vi "Utility - Configuration File Generator.vi"() -> ()   [LabVIEW 2013]
uses:
  controls/TDMS Properties.ctl
  controls/Acquisition and Logging Configuration.ctl
  <vilib>/Utility/xml.llb/Write to XML File(string).vi
panel:
  in  "Enable Time Trigger":bool caption="启用时间触发"
  in  "Enable RMS Trigger":bool=TRUE caption="启用RMS触发"
  in  "Log Continuously":bool caption="连续记录"
  in  "TDMS Properties":T1[](array[typedef])=[{"Name"="公司", "Value"="[公司名称]"}, {"Name"="作者(author)", "Value"="[开发者姓名]"}, {"Name"="运算符", "Value"="[操作员名]"}, {"Name"="测试系统", "Value"="[系统名]"}, {"Name"="位置", "Value"="[位置]"}, {"Name"="线", "Value"="[行]"}, {"Name"="机器", "Value"="[机器名]"}, {"Name"="说明", "Value"="[说明]"}] caption="TDMS属性"
  in  "Trigger - Time (Minute)":i32=30 caption="触发－时间（分钟）"
  in  "Trigger - Channel":i32 caption="触发－通道"
  in  "Trigger - RMS Value":dbl=2.0 caption="触发－均方根值"
  in  "Channel Names":string[](array[string])=["Dev1/ai0", "Dev1/ai1", "Dev1/ai2", "Dev1/ai3"] caption="通道名"
  in  "Channel Scale Array":dbl[](array[numeric])=[1.0, 1.0, 1.0, 1.0] caption="通道换算数组"
  in  "Number of Channels":i32=4 caption="通道数"
  in  "Data File Name":string="DAQ_数据" caption="数据文件名"
  in  "Number of Reads to Save":i32=20 caption="用于保存的读取次数"
  in  "Samples per Read":i32=1000 caption="每次读取采样"
  in  "Data Rate (Hz)":dbl=1000.0 caption="数据率(Hz)"
  # "操作步骤：为下列控件赋值，然后运行VI，在项目的根目录中生成Config.xml文件。\n\n注：生成Config.xml以后，需将其复制至RT终端根目录中。"
  # "采集"
  # "通道"
  # "记录"
  # "触发"
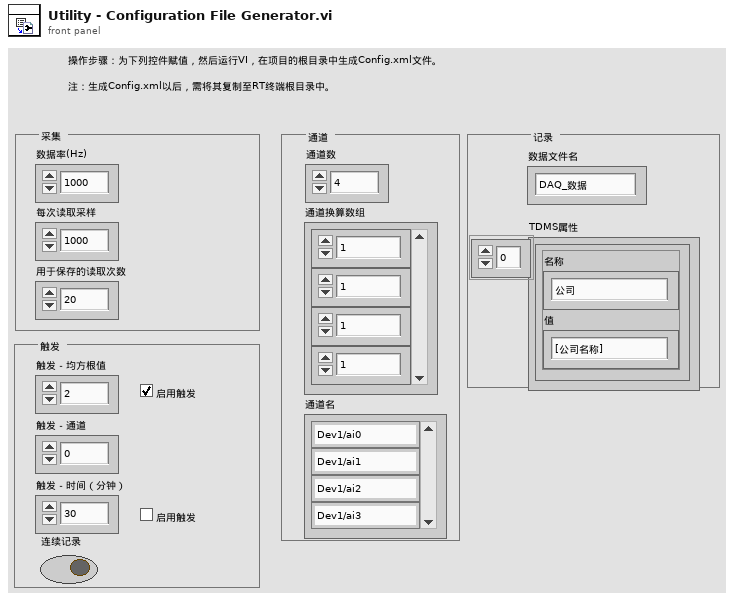
[diagram p1: front panel]
types:
  T1 = typedef "TDMS Properties.ctl" = cluster{"Name":string, "Value":string}
  T2 = typedef "Acquisition and Logging Configuration.ctl" = cluster{"Data Rate (Hz)":dbl, "Samples per Read":i32, "Number of Reads to Save":i32, "Data File Name":string, "TDMS Properties":T1[], "Number of Channels":i32, "Channel Scale Array":dbl[], "Channel Names":string[], "Trigger - RMS Value":dbl, "Trigger - Channel":i32, "Trigger - Time (Minute)":i32, "Enable RMS Trigger":bool, "Enable Time Trigger":bool, "Always Log":bool}
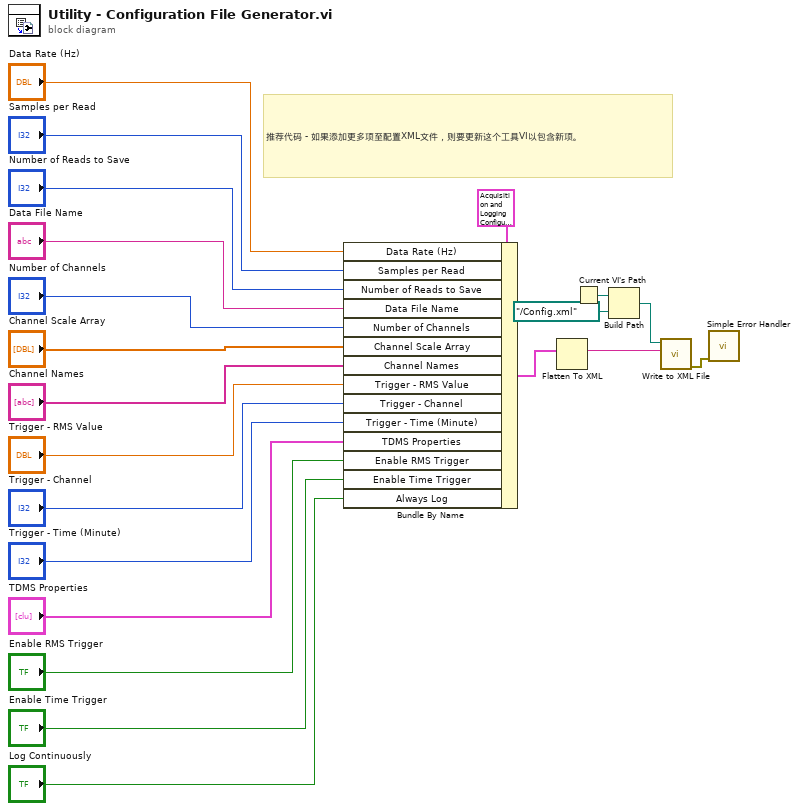
[diagram p0: block diagram]
diagram:
  # "推荐代码 - 如果添加更多项至配置XML文件，则要更新这个工具VI以包含新项。"
  n1 = Bundle By Name(cluster=T2 {"Data Rate (Hz)"=1.0, "Samples per Read"=0, "Number of Reads to Save"=0, "Data File Name"="", "TDMS Properties"=[], "Number of Channels"=0, "Channel Scale Array"=[0.0, 0.0, 0.0, 0.0], "Channel Names"=[], "Trigger - RMS Value"=0.0, "Trigger - Channel"=0, "Trigger - Time (Minute)"=0, "Enable RMS Trigger"=FALSE, "Enable Time Trigger"=FALSE, "Always Log"=FALSE} ("Acquisition and Logging Configuration"), "Data Rate (Hz)"="Data Rate (Hz)", "Samples per Read"="Samples per Read", "Number of Reads to Save"="Number of Reads to Save", "Data File Name"="Data File Name", "Number of Channels"="Number of Channels", "Channel Scale Array"="Channel Scale Array", "Channel Names"="Channel Names", "Trigger - RMS Value"="Trigger - RMS Value", "Trigger - Channel"="Trigger - Channel", "Trigger - Time (Minute)"="Trigger - Time (Minute)", "TDMS Properties"="TDMS Properties", "Enable RMS Trigger"="Enable RMS Trigger", "Enable Time Trigger"="Enable Time Trigger", "Always Log"="Log Continuously") -> (w20:T2)
  n2 = Flatten To XML(anything=w20) -> (xml string=w19:string)
  n3 = Current VI's Path() -> (path=w18:path)
  n4 = Build Path(base path=w18, name or relative path=path "../Config.xml") -> (appended path=w16:path)
  n5 = call-poly <vilib>:"Write to XML File.vi"("XML Input"=w19, "XML File Path"=w16) -> ("error out"=w15:errorcluster)  [unwired: 7 in, 2 out]
  n6 = call <vilib>:"Simple Error Handler.vi"("error in (no error)"=w15) -> ()  [unwired: 4 in, 5 out]
